vi "LJUD_OpenLabJackS.vi"(6 "FirstFound":bool=TRUE, 7 "Address":string="192.168.1.209", 8 "error in":errorcluster, 9 "ConnectionType":string="LJ_ctUSB", 10 "DeviceType":string="LJ_dtUE9") -> (0 "error out":errorcluster, 1 "warning out":errorcluster, 3 "Handle":i32)   [LabVIEW 2019]
doc: "Call an Open function to get a handle to a device. That handle\nis then passed to other functions to write & read values.\n\nDocumented in Section 4.2 of the device's datasheet, with further\ninformation in Section 4.3.\n\nDeviceType: LJ_dtU3=3, LJ_dtU6=6, LJ_dtUE9=9\n\nConnectionType: LJ_ctUSB=1, LJ_ctETHERNET=2\n\nAddress: For USB, pass the local ID or serial number of the desired\nLabJack. For Ethernet pass the IP address of the desired LabJack. If\nFirstFound is true, Address is ignored.\n\nFirstFound: If true, then the Address and ConnectionType parameters\nare ignored and the driver opens the first LabJack found with the\nspecified DeviceType. Generally only recommended when a single\nLabJack is connected. Currently only supported with USB. If a USB\ndevice is not found, it will try Ethernet but with the given Address."
uses:
  labjackud.dll
panel:
  # "Call an Open function to get a handle to a device.  That handle\nis then passed to other functions to write & read values.\n\nDocumented in Section 4.2 of the device's datasheet, with further\ninformation in Section 4.3.\n\nDeviceType:  LJ_dtU3=3, LJ_dtU6=6, LJ_dtUE9=9\n\nConnectionType:  LJ_ctUSB=1, LJ_ctETHERNET=2\n\nAddress:  For USB, pass the local ID or serial number of the desired\nLabJack. For Ethernet pass the IP address of the desired LabJack. If\nFirstFound is true, Address is ignored.\n\nFirstFound:  If true, then the Address and ConnectionType parameters\nare ignored and the driver opens the first LabJack found with the\nspecified DeviceType. Generally only recommended when a single\nLabJack is connected. Currently only supported with USB. If a USB\ndevice is not found, it will try Ethernet but with the given Address."
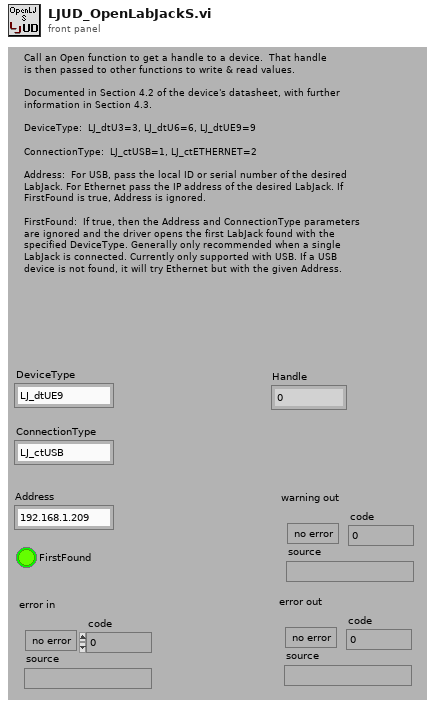
[diagram p1: front panel]
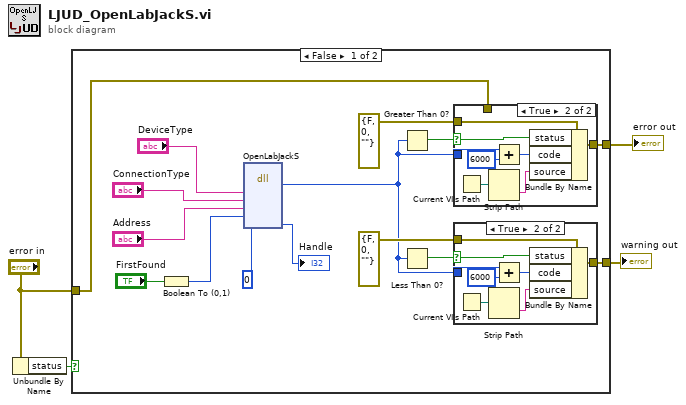
[diagram p0: block diagram]
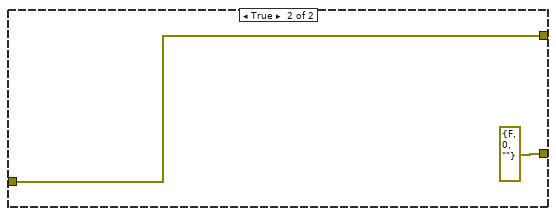
[diagram p4: hidden frame]
diagram:
  n1 = Unbundle By Name("error in") -> ("status"=w2:bool)
  n2 = case shown="False" w2 {
    tunnel: [w10 w38] -> w4
    tunnel: [w6 errorcluster {"status"=FALSE, "code"=0, "source"=""} ("error IO")] -> w3
    tunnel: "error in" -> [w5 w38]
    frame False {
      n3 = Boolean To (0,1)(Boolean="FirstFound") -> (0, 1=w15:i16)
      n4 = dll-call lib="labjackud.dll" fn="OpenLabJackS"("DeviceType"="DeviceType", "ConnectionType"="ConnectionType", "Address"="Address", "FirstFound"=w15, "Handle"=0) -> (w7:i32, "Handle"=→"Handle":i32)  [unwired: 7 in, 2 out]
      n5 = Greater Than 0?(x=w7) -> (x > 0?=w11:bool)
      n6 = Less Than 0?(x=w7) -> (x < 0?=w9:bool)
      n7 = case shown="True" w11 {
        selector: w11 -> [_ w36]
        tunnel: [w29 w37] -> w10
        tunnel: errorcluster {"status"=FALSE, "code"=0, "source"=""} ("error IO") -> [_ w35]
        tunnel: w7 -> [_ w31]
        tunnel: w5 -> [w29 _]
        frame False {
        }
        frame True {
          n8 = Current VI's Path() -> (path=w33:path)
          n9 = Strip Path(path=w33) -> (name=w34:string)  [unwired: 1 out]
          n10 = Add(x=w31, y=6000) -> (x+y=w32:i32)
          n11 = Bundle By Name(cluster=w35, "status"=w36, "code"=w32, "source"=w34) -> (w37:errorcluster)
        }
      }
      n12 = case shown="True" w9 {
        selector: w9 -> [_ w27]
        tunnel: [w20 w28] -> w6
        tunnel: errorcluster {"status"=FALSE, "code"=0, "source"=""} ("error IO") -> [w20 w26]
        tunnel: w7 -> [_ w22]
        frame False {
        }
        frame True {
          n13 = Current VI's Path() -> (path=w24:path)
          n14 = Strip Path(path=w24) -> (name=w25:string)  [unwired: 1 out]
          n15 = Add(x=w22, y=6000) -> (x+y=w23:i32)
          n16 = Bundle By Name(cluster=w26, "status"=w27, "code"=w23, "source"=w25) -> (w28:errorcluster)
        }
      }
    }
    frame True {
    }
  }
  "error out" <- w4
  "warning out" <- w3
